vi "Gruppen sichtbar schalten.vi"(0 "Element Referenzen":refnum<vi>[](array[refnum]), 7 "Sichtbar":bool, 11 "error in (no error)":errorcluster caption="Fehler (Eingang, kein Fehler)") -> (15 "error out":errorcluster caption="Fehler (Ausgang)")   [LabVIEW 2020, in "Anlagenuebersicht.lvlib" / "VisBx Anzeige.lvlib"]
uses:
  VisBx Anzeige.lvlib
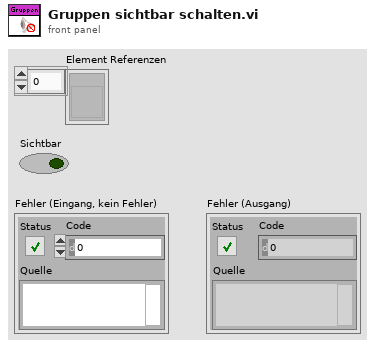
[diagram p1: front panel]
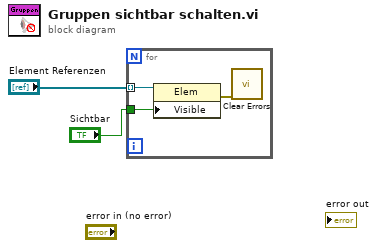
[diagram p0: block diagram]
diagram:
  n1 = for {
    tunnel: "Element Referenzen" -> [w5] mode=indexing
    tunnel: "Sichtbar" -> [w3]
    n2 = property class="Elem"(reference=w5, "Visible"=w3) -> (error out=w4:errorcluster)  [unwired: 1 in, 1 out]
    n3 = call <vilib>:"Clear Errors.vi"("error in (no error)"=w4) -> ()  [unwired: 5 in, 2 out]
  }
